vi "visa test.vi"(11 "VISA resource name":refnum<visa-resource-name>="COM3") -> (0 "MB Address":i32, 1 "Parity":u16, 2 "Baud Rate":u32, 3 "find?":bool)   [LabVIEW 2020]
uses:
  <vilib>/NI Modbus.llb/MB Serial Master Query Read Holding Registers (poly).vi
panel:
  in  "Cancel button":bool
  out "Slide":i32(slide) scale=0.0..3458.0
  out "String":string
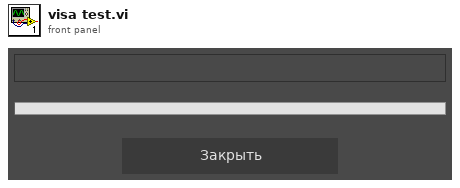
[diagram p1: front panel]
types:
  T1 = cluster{"Mode":enum16{"RTU", "ASCII"}, "Slave Address":u8}
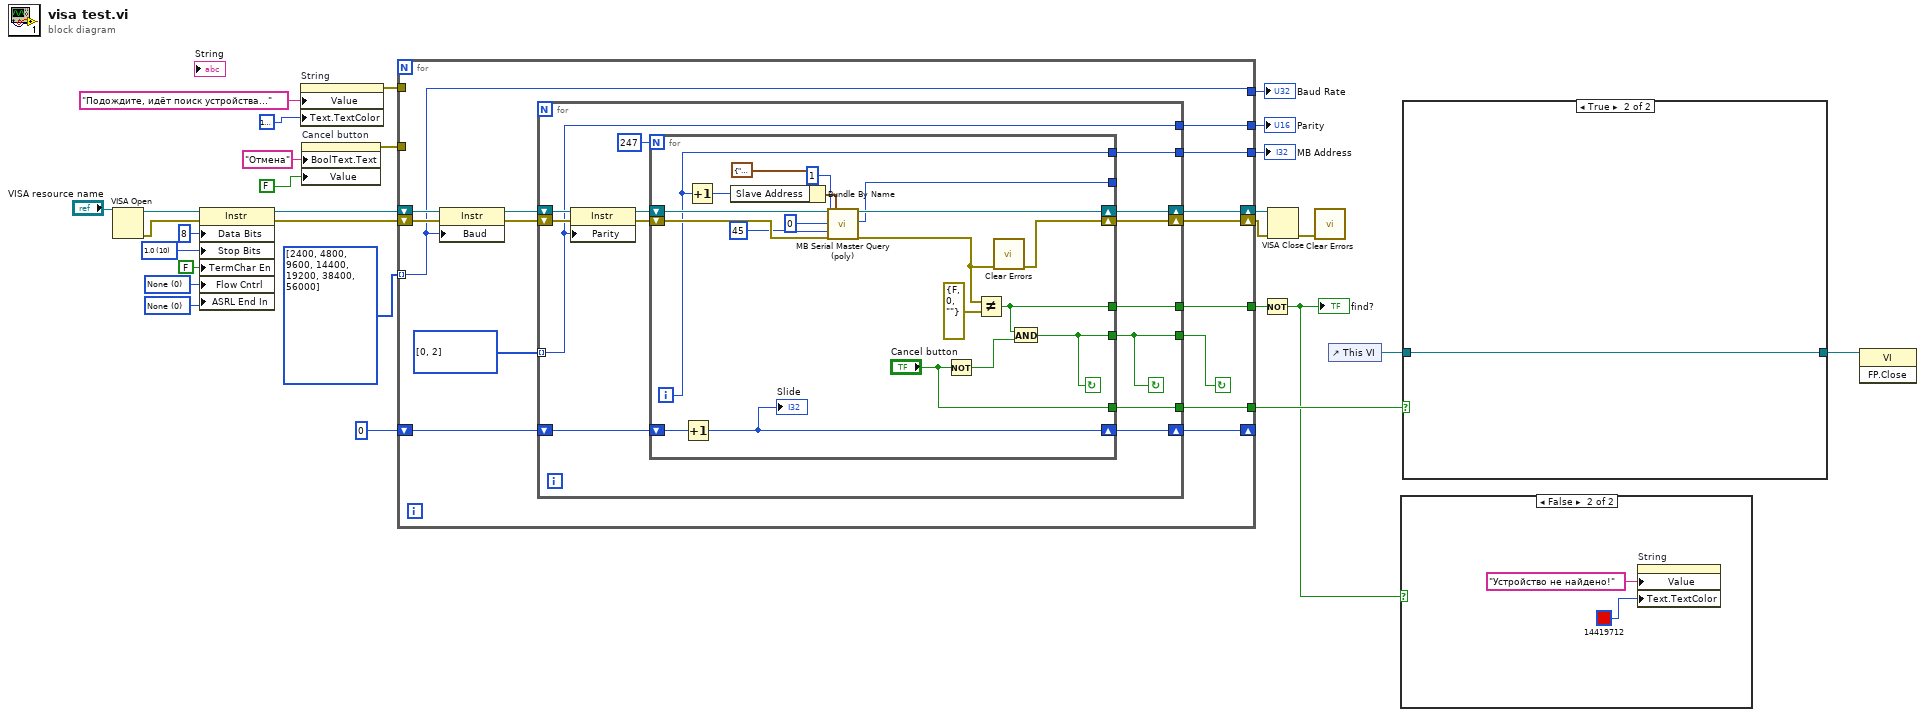
[diagram p0: block diagram]
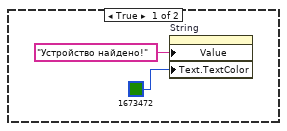
[diagram p2: hidden frame]
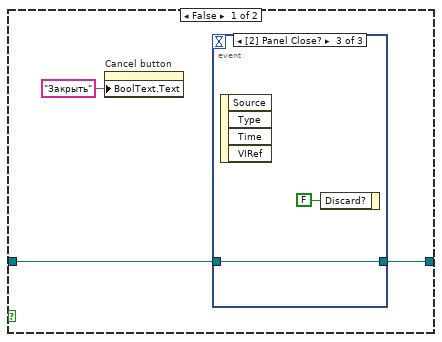
[diagram p3: hidden frame]
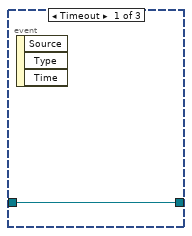
[diagram p4: hidden frame]
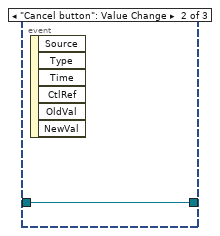
[diagram p5: hidden frame]
diagram:
  w16 = u16 0 items=["None", "Last Bit", "TermChar"] ("Serial Settings:End Mode for Reads")
  w17 = u16 0 items=["None", "XON/XOFF", "RTS/CTS", "XON/XOFF & RTS/CTS", "DTR/DSR", "XON/XOFF & DTR/DSR"] ("Serial Settings:Flow Control")
  w19 = u16 10 items=["1.0"=10, "1.5"=15, "2.0"=20] ("Serial Settings:Stop Bits")
  n1 = VISA Open(VISA resource name="VISA resource name") -> (VISA resource name=w22:refnum<visa-resource-name>, error out=w21:errorcluster)  [unwired: 4 in]
  n2 = property class="Instr"(reference=w22, error in=w21, "Data Bits"=u16 8 ("Serial Settings:Data Bits"), "Stop Bits"=w19, "TermChar En"=FALSE ("Message Based Settings:Termination Character Enable"), "Flow Cntrl"=w17, "ASRL End In"=w16) -> (reference out=w15:refnum<visa-resource-name>, error out=w14:errorcluster)
  n3 = property on="String" class="Str"("Value"="Подождите, идёт поиск устройства..." ("String"), "Text.TextColor"=u32 16777238) -> (error out=w9:errorcluster)  [unwired: 2 in, 1 out]
  n4 = property on="Cancel button" class="Bool (strict)"("BoolText.Text"="Отмена" ("Boolean Text.Text"), "Value"=FALSE ("Cancel button")) -> (error out=w3:errorcluster)  [unwired: 2 in, 1 out]
  n5 = for {
    tunnel: u32[] [2400, 4800, 9600, 14400, 19200, 38400, 56000] -> [w40] mode=indexing
    tunnel: [w40] -> w25
    tunnel: [w39] -> w24
    tunnel: [w38] -> w23
    shift-right: [w37] -> w27
    shift-left: w15 -> [w44]
    shift-right: [w36] -> w28
    shift-left: w14 -> [w43]
    tunnel: [w30] -> w26
    shift-right: [w32] -> _
    shift-left: 0 -> [w33]
    tunnel: w9 -> [_]
    tunnel: [w31] -> w8
    tunnel: w3 -> [_]
    stop <- w35 continue-if-true
    w34 = u16[] [0, 2] items=["None", "Odd", "Even", "Mark", "Space"]
    n6 = property class="Instr"(reference=w44, error in=w43, "Baud"=w40) -> (reference out=w42:refnum<visa-resource-name>, error out=w41:errorcluster)
    n7 = for {
      tunnel: w34 -> [w50] mode=indexing
      shift-right: [w53] -> w37
      shift-left: w42 -> [w58]
      shift-right: [w52] -> w36
      shift-left: w41 -> [w57]
      tunnel: [w51] -> w38
      tunnel: [w50] -> w39
      tunnel: [w49] -> w35
      shift-right: [w47] -> w32
      shift-left: w33 -> [w48]
      tunnel: [w46] -> w31
      tunnel: [w45] -> w30
      stop <- w49 continue-if-true
      n8 = property class="Instr"(reference=w58, error in=w57, "Parity"=w50) -> (reference out=w55:refnum<visa-resource-name>, error out=w54:errorcluster)
      n9 = for {
        N: 247 -> [_]
        tunnel: [w60] -> w49
        shift-right: [w72] -> w52
        shift-left: w54 -> [w77]
        shift-right: [w71] -> w53
        shift-left: w55 -> [w78]
        tunnel: [w69] -> w51
        tunnel: [w66] -> _
        shift-right: [w62] -> w47
        shift-left: w48 -> [w63]
        tunnel: ["Cancel button"] -> w46
        tunnel: [w59] -> w45
        i -> [w69]
        stop <- w60 continue-if-true
        n10 = Increment(x=w63) -> (x+1=w62:i32)
        "Slide" <- w62
        n11 = Increment(x=w69) -> (x+1=w70:i32)
        n12 = Bundle By Name(cluster=T1 {"Mode"=enum."RTU", "Slave Address"=0} ("Serial Parameters"), "Slave Address"=w70) -> (w75:T1)
        n13 = call-poly <vilib>:"MB Serial Master Query (poly).vi"("VISA resource name"=w78, "Starting Address"=u16 0, "Quantity"=u16 1, "Timeout"=u32 45, "error in"=w77, "Serial Parameters"=w75) -> ("VISA resource name out"=w71:refnum<visa-resource-name>, "Exception Code"=w66:u8, "error out"=w68:errorcluster)  [unwired: 10 in, 1 out]
        n14 = Not(x="Cancel button") -> (.not. x?=w64:bool)
        n15 = Not Equal?(x=w68, y=errorcluster {"status"=FALSE, "code"=0, "source"=""}) -> (x != y?=w59:bool)
        n16 = call <vilib>:"Clear Errors.vi"("error in (no error)"=w68) -> ("error out"=w72:errorcluster)  [unwired: 5 in, 1 out]
        n17 = And(x=w59, y=w64) -> (x .and. y?=w60:bool)
      }
    }
  }
  "Baud Rate" <- w25
  "Parity" <- w24
  "MB Address" <- w23
  n18 = Not(x=w26) -> (.not. x?=w7:bool)
  "find?" <- w7
  n19 = VISA Close(VISA resource name=w27, error in (no error)=w28) -> (error out=w2:errorcluster)
  n20 = call <vilib>:"Clear Errors.vi"("error in (no error)"=w2) -> ()  [unwired: 5 in, 2 out]
  n21 = control-ref of="This VI"() -> (w6:refnum<vi>)
  n22 = case shown="False" w7 {
    frame True {
      n23 = property on="String" class="Str"("Value"="Устройство найдено!" ("String"), "Text.TextColor"=u32 1673472) -> ()  [unwired: 2 in, 2 out]
    }
    frame False {
      n24 = property on="String" class="Str"("Value"="Устройство не найдено!" ("String"), "Text.TextColor"=u32 14419712) -> ()  [unwired: 2 in, 2 out]
    }
  }
  n25 = case shown="True" w8 {
    tunnel: [w83 w90] -> w5
    tunnel: w6 -> [w84 w90]
    frame False {
      n26 = property on="Cancel button" class="Bool (strict)"("BoolText.Text"="Закрыть" ("Boolean Text.Text")) -> ()  [unwired: 2 in, 2 out]
      n27 = event shown="[2] Panel Close?" {
        selector: _ -> [_ _ _]
        dyn-events: _ -> [_ _ _]
        timeout: _ -> [_ _ _]
        tunnel: w84 -> [w86 w87 w88]
        tunnel: [w86 w87 w88] -> w83
        event Timeout {
          n28 = event-data() -> ()  [unwired: 1 in, 3 out]
        }
        event "Cancel button": Value Change {
          n29 = event-data() -> ()  [unwired: 1 in, 6 out]
        }
        event Panel Close? {
          n30 = event-data() -> ()  [unwired: 1 in, 4 out]
          n31 = event-data("Discard?"=FALSE) -> ()  [unwired: 1 in, 1 out]
        }
      }
    }
    frame True {
    }
  }
  n32 = invoke class="VI" method="FP.Close"(reference=w5) -> ()  [unwired: 2 in, 3 out]
